vi "Variant To String.vi"(7 "Variant":variant) -> (8 "String":string, 15 "Data Type":string)   [LabVIEW 2017, in "TreeLUT.lvclass"]
uses:
  TreeLUT.lvclass
  <vilib>/Utility/Data Type/NI_Data Type.lvlib
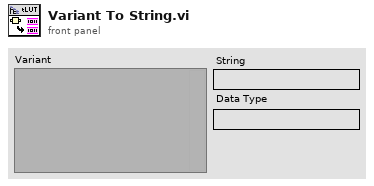
[diagram p1: front panel]
types:
  T1 = typedef "NI_Data Type.lvlib/Data Type.ctl" = enum8{"Invalid Type", "Void", "I8", "I16", "I32", "I64", "U8", "U16", "U32", "U64", "Single Float", "Double Float", "Extended Float", "Single Complex", "Double Complex", "Extended Complex", "Enum U8", "Enum U16", "Enum U32", "Enum U64", "Single Float With Unit", "Double Float With Unit", "Extended Float With Unit", "Single Complex with Unit", "Double Complex with Unit", "Extended Complex with Unit", "Boolean", "String", "Path", "Picture", "Tag", "Array", "Cluster", "Variant", "LV Variant", "Waveform", "Timestamp", "Digital Waveform", "Digital Data", "ExpressData", "Refnum", "External Data", "VI", "Poly VI", "LabVIEW Class Instance", "Fixed Point"}
  T2 = typedef "NI_Data Type.lvlib/Type Definition Info.ctl" = cluster{"Name":string, "Timestamp":u32}
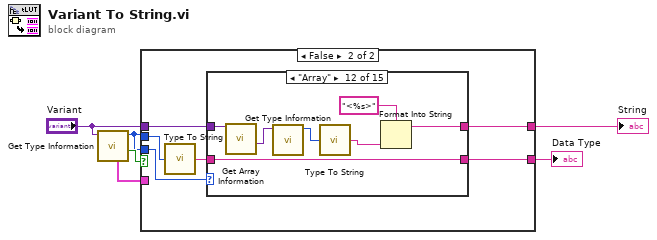
[diagram p0: block diagram]
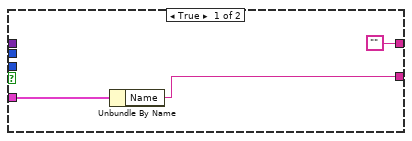
[diagram p2: hidden frame]
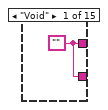
[diagram p3: hidden frame]
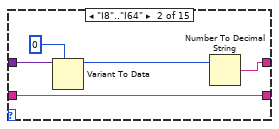
[diagram p4: hidden frame]
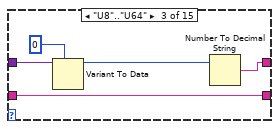
[diagram p5: hidden frame]
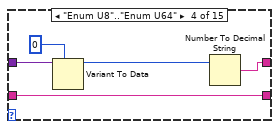
[diagram p6: hidden frame]
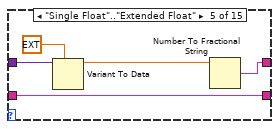
[diagram p7: hidden frame]
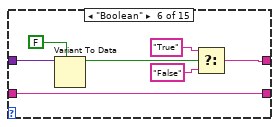
[diagram p8: hidden frame]
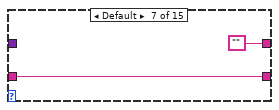
[diagram p9: hidden frame]
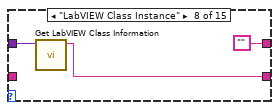
[diagram p10: hidden frame]
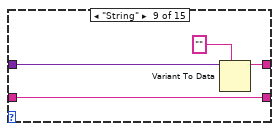
[diagram p11: hidden frame]
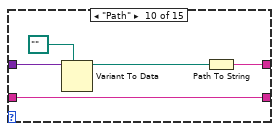
[diagram p12: hidden frame]
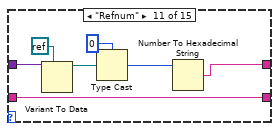
[diagram p13: hidden frame]
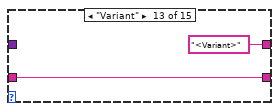
[diagram p14: hidden frame]
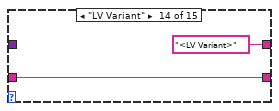
[diagram p15: hidden frame]
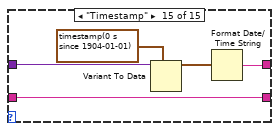
[diagram p16: hidden frame]
diagram:
  n1 = call <vilib>:"Get Type Information.vi"("Variant"="Variant") -> ("Type Definition"=w4:bool, "Type"=w1:T1, "Type Definition Info"=w3:T2)  [unwired: 6 in, 2 out]
  n2 = case shown="False" w4 {
    tunnel: w1 -> [_ w13]
    tunnel: "Variant" -> [_ w15]
    tunnel: ["" w14] -> w5
    tunnel: w3 -> [w9 _]
    tunnel: [w8 w11] -> w2
    tunnel: w1 -> [_ w12]
    frame True {
      n3 = Unbundle By Name(w9) -> ("Name"=w8:string)
    }
    frame False {
      n4 = call "Type To String.vi"("Data Type"=w12) -> ("Data Type String"=w10:string)  [unwired: 14 in]
      n5 = case shown="\"Array\"" w13 {
        tunnel: w15 -> [_ w21 w26 w31 w36 w43 _ w47 w52 w57 w63 w70 _ _ w80]
        tunnel: [w16 w18 w23 w28 w33 w38 "" "" w50 w54 w58 w65 "<Variant>" ("f") "<LV Variant>" ("f") w76] -> w14
        tunnel: [w16 w17 w22 w27 w32 w37 w45 w46 w49 w53 w64 w71 w72 w74 w78] -> w11
        tunnel: w10 -> [_ w17 w22 w27 w32 w37 w45 _ w49 w53 w64 w71 w72 w74 w78]
        frame "Void" {
          w16 = ""
        }
        frame "I8".."I64" {
          n6 = Variant To Data(type=i64 0, Variant=w21) -> (data=w19:i64)  [unwired: 1 in, 1 out]
          n7 = Number To Decimal String(number=w19) -> (decimal integer string=w18:string)  [unwired: 1 in]
        }
        frame "U8".."U64" {
          n8 = Variant To Data(type=u64 0, Variant=w26) -> (data=w25:u64)  [unwired: 1 in, 1 out]
          n9 = Number To Decimal String(number=w25) -> (decimal integer string=w23:string)  [unwired: 1 in]
        }
        frame "Enum U8".."Enum U64" {
          n10 = Variant To Data(type=u64 0, Variant=w31) -> (data=w29:u64)  [unwired: 1 in, 1 out]
          n11 = Number To Decimal String(number=w29) -> (decimal integer string=w28:string)  [unwired: 1 in]
        }
        frame "Single Float".."Extended Float" {
          n12 = Variant To Data(type=ext 0.0, Variant=w36) -> (data=w34:ext)  [unwired: 1 in, 1 out]
          n13 = Number To Fractional String(number=w34) -> (F-format string=w33:string)  [unwired: 3 in]
        }
        frame "Boolean" {
          n14 = Variant To Data(type=FALSE, Variant=w43) -> (data=w41:bool)  [unwired: 1 in, 1 out]
          n15 = Select(t="True", s=w41, f="False") -> (s? t:f=w38:string)
        }
        frame Default {
        }
        frame "LabVIEW Class Instance" {
          n16 = call <vilib>:"Get LabVIEW Class Information.vi"("Variant"=w47) -> ("LabVIEW Class File Name"=w46:string)  [unwired: 8 in, 2 out]
        }
        frame "String" {
          n17 = Variant To Data(type="", Variant=w52) -> (data=w50:string)  [unwired: 1 in, 1 out]
        }
        frame "Path" {
          n18 = Variant To Data(type=path "", Variant=w57) -> (data=w55:path)  [unwired: 1 in, 1 out]
          n19 = Path To String(path=w55) -> (string=w54:string)
        }
        frame "Refnum" {
          n20 = Variant To Data(type=refnum<k0> refnum, Variant=w63) -> (data=w61:refnum<k0>)  [unwired: 1 in, 1 out]
          n21 = Type Cast(type=0, x=w61) -> (*(type *) &x=w59:i32)
          n22 = Number To Hexadecimal String(2:w59) -> (0:w58:string)  [unwired: 1 in]
        }
        frame "Array" {
          n23 = call <vilib>:"Get Array Information.vi"("Variant"=w70) -> ("Array Element Data Type"=w69:variant)  [unwired: 7 in, 3 out]
          n24 = call <vilib>:"Get Type Information.vi"("Variant"=w69) -> ("Type"=w68:T1)  [unwired: 6 in, 4 out]
          n25 = call "Type To String.vi"("Data Type"=w68) -> ("Data Type String"=w66:string)  [unwired: 14 in]
          n26 = Format Into String(format string="<%s>", w66) -> (resulting string=w65:string)  [unwired: 2 in, 1 out]
        }
        frame "Variant" {
        }
        frame "LV Variant" {
        }
        frame "Timestamp" {
          n27 = Variant To Data(type=timestamp(0 s since 1904-01-01), Variant=w80) -> (data=w77:timestamp)  [unwired: 1 in, 1 out]
          n28 = Format Date/Time String(seconds (now)=w77) -> (date/time string=w76:string)  [unwired: 2 in]
        }
      }
    }
  }
  "String" <- w5
  "Data Type" <- w2
